vi "rtPressure.vi"(9 "Pressure Out (mA)":dbl, 10 "Pressure In (mA)":dbl) -> (0 "Delta Pressure (psi)":dbl, 1 "Pressure Out (psi)":dbl, 2 "Pressure In (psi)":dbl)   [LabVIEW 2019]
panel:
  # "Rotary Pressure"
  # "Honeywell MLH08KPSB01B"
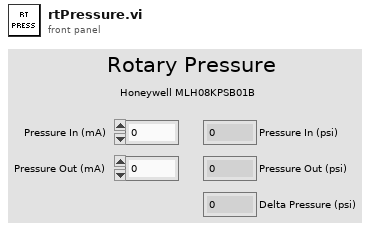
[diagram p1: front panel]
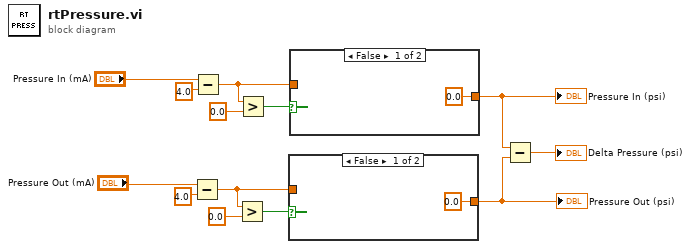
[diagram p0: block diagram]
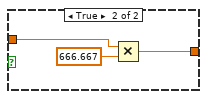
[diagram p2: hidden frame]
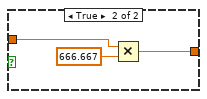
[diagram p3: hidden frame]
diagram:
  n1 = Subtract(x="Pressure Out (mA)", y=4.0) -> (x-y=w3:dbl)
  n2 = Subtract(x="Pressure In (mA)", y=4.0) -> (x-y=w8:dbl)
  n3 = Greater?(x=w3, y=0.0) -> (0:w5:bool)
  n4 = Greater?(x=w8, y=0.0) -> (0:w10:bool)
  n5 = case shown="False" w5 {
    tunnel: w3 -> [_ w16]
    tunnel: [0.0 w15] -> w2
    frame False {
    }
    frame True {
      n6 = Multiply(x=w16, y=666.667) -> (x*y=w15:dbl)
    }
  }
  "Pressure Out (psi)" <- w2
  n7 = case shown="False" w10 {
    tunnel: w8 -> [_ w20]
    tunnel: [0.0 w19] -> w7
    frame False {
    }
    frame True {
      n8 = Multiply(x=w20, y=666.667) -> (x*y=w19:dbl)
    }
  }
  "Pressure In (psi)" <- w7
  n9 = Subtract(x=w7, y=w2) -> (x-y=→"Delta Pressure (psi)":dbl)
